vi "MCL Init Handle.vi"() -> (3 "function return":i32)   [LabVIEW 2017, in "Madlib.lvlib"]
doc: "MADLIB_API int MCL_InitHandle();"
uses:
  Madlib.lvlib
  Madlib.dll
panel:
  out "error out":errorcluster
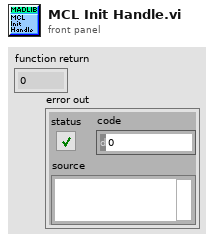
[diagram p1: front panel]
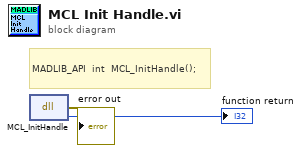
[diagram p0: block diagram]
diagram:
  # "MADLIB_API  int\t\tMCL_InitHandle();"
  n1 = dll-call lib="C:/Users/Fred/dev/pump-probe/Piezo/lvlib/Madlib.*" fn="MCL_InitHandle"() -> (error out=→"error out":errorcluster, →"function return":i32)  [unwired: 3 in, 1 out]
